vi "local_linear_smooth_double_.vi"(1 "Smoothing Parameter (Gaussian S.D. in pixels)":dbl=3.0, 2 "Input Array":dbl[][](graph)=array100x100[10000 elements]) -> (0 "Smoothed Array":dbl[][](graph))   [LabVIEW 2020]
uses:
  <vilib>/Analysis/baseanly.llb/Real A x B.vi
  <vilib>/Analysis/NI_AALBase.lvlib
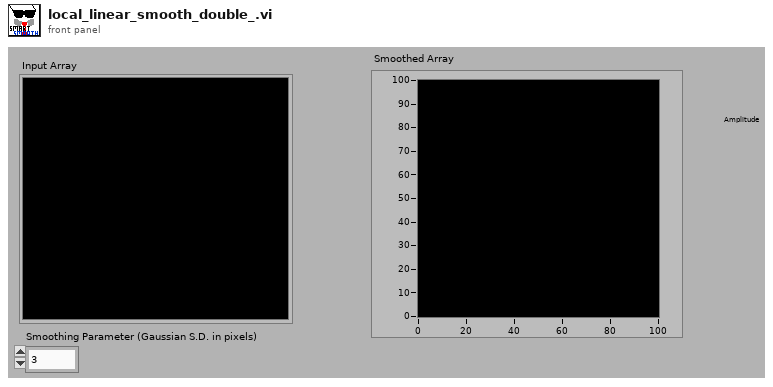
[diagram p1: front panel]
types:
  T1 = typedef "NI_Matrix.lvlib/RealMatrix.ctl" = dbl[][]
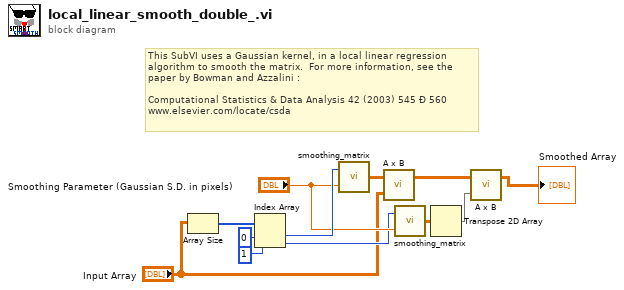
[diagram p0: block diagram]
diagram:
  # "This SubVI uses a Gaussian kernel, in a local linear regression algorithm to smooth the matrix.  For more information, see the paper by Bowman and Azzalini :\n\nComputational Statistics & Data Analysis 42 (2003) 545 Ð 560 \nwww.elsevier.com/locate/csda"
  n1 = Array Size(array="Input Array") -> (size(s)=w9:i32[])
  n2 = Index Array(array=w9, index #1=0 ("index"), index #2=1 ("index")) -> (element #1=w6:i32, element #2=w3:i32)
  n3 = call "smoothing_matrix.vi"("Smoothing Parameter (Gaussian S.D. in pixels)"="Smoothing Parameter (Gaussian S.D. in pixels)", "Size"=w6) -> ("Smoothing Matrix"=w12:dbl[][])
  n4 = call-poly <vilib>:"A x B.vi"("B"="Input Array", "A"=w12) -> ("A x B"=w11:T1)  [unwired: 1 out]
  n5 = call "smoothing_matrix.vi"("Smoothing Parameter (Gaussian S.D. in pixels)"="Smoothing Parameter (Gaussian S.D. in pixels)", "Size"=w3) -> ("Smoothing Matrix"=w5:dbl[][])
  n6 = Transpose 2D Array(2D array=w5) -> (transposed array=w10:dbl[][])
  n7 = call-poly <vilib>:"A x B.vi"("B"=w10, "A"=w11) -> ("A x B"=→"Smoothed Array":T1)  [unwired: 1 out]
